vi "Filter Unmarked Lines.vi"(6 "Ignore Empty Cell?":bool=TRUE, 8 "error in (no error)":errorcluster, 9 "unmarked RegExp":string="^[*^]+$", 10 "Col Index":i32, 11 "CfgTable in":string[][](array[string])) -> (0 "error out":errorcluster, 3 "CfgTable out":string[][](array[string]))   [LabVIEW 2017, in "ClusterCfgTable.lvlib"]
uses:
  ClusterCfgTable.lvlib
  <userlib>/_OpenG.lib/string/string.llb/Trim Whitespace (String)__ogtk.vi
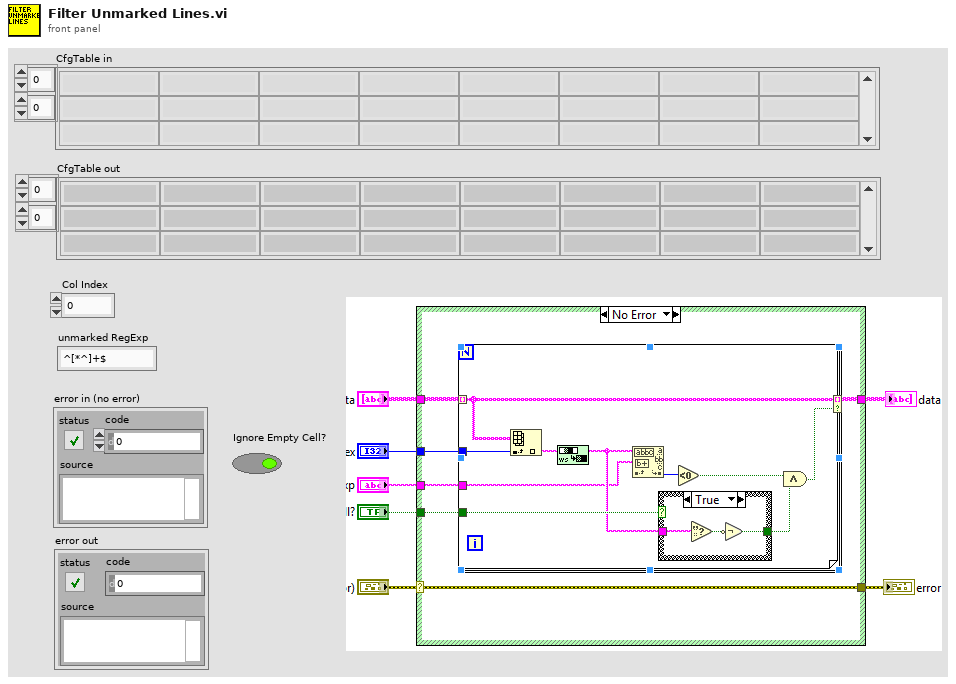
[diagram p1: front panel]
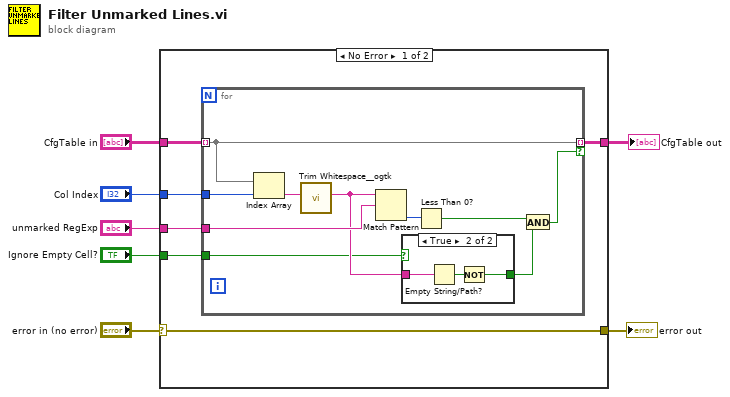
[diagram p0: block diagram]
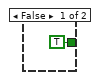
[diagram p2: hidden frame]
diagram:
  n1 = case shown="No Error" "error in (no error)" {
    selector: "error in (no error)" -> [w8 w29]
    tunnel: "Col Index" -> [w13 _]
    tunnel: [w12 w28] -> w6
    tunnel: "CfgTable in" -> [w11 w28]
    tunnel: "unmarked RegExp" -> [w10 _]
    tunnel: "Ignore Empty Cell?" -> [w9 _]
    tunnel: [w8 w29] -> w1
    frame No Error {
      n2 = for {
        tunnel: w11 -> [w23] mode=indexing
        tunnel: [w23] -> w12 mode=indexing if=w17
        tunnel: w13 -> [w22]
        tunnel: w10 -> [w19]
        tunnel: w9 -> [w14]
        n3 = Index Array(array=w23, index=w22) -> (element=w20:string)
        n4 = call-poly <userlib>:"Trim Whitespace__ogtk.vi"("String in"=w20) -> ("String out"=w18:string)  [unwired: 6 in]
        n5 = Match Pattern(string=w18, regular expression=w19) -> (offset past match=w21:i32)  [unwired: 1 in, 3 out]
        n6 = case shown="True" w14 {
          tunnel: w18 -> [_ w27]
          tunnel: [TRUE w25] -> w15
          frame False {
          }
          frame True {
            n7 = Empty String/Path?(string/path=w27) -> (empty?=w26:bool)
            n8 = Not(x=w26) -> (.not. x?=w25:bool)
          }
        }
        n9 = Less Than 0?(x=w21) -> (x < 0?=w16:bool)
        n10 = And(x=w16, y=w15) -> (x .and. y?=w17:bool)
      }
    }
    frame Error {
    }
  }
  "error out" <- w1
  "CfgTable out" <- w6
